vi "apply.vi"(8 "error in (no error)":errorcluster caption="entrée d'erreur (pas d'erreur)", 11 "Tree.lvclass 2":refnum<class "Tree.lvclass">) -> (0 "error out":errorcluster caption="sortie d'erreur", 2 "X_leaves":dbl[][](array[numeric]), 3 "Tree.lvclass":refnum<class "Tree.lvclass">)   [LabVIEW 2020, in "Tree.lvclass"]
doc: "Return the index of the leaf that each sample is predicted as.\n\n .. versionadded:: 0.17\n\n Parameters\n ----------\n X : {array-like, sparse matrix} of shape (n_samples, n_features)\n The input samples. Internally, it will be converted to\n ``dtype=np.float32`` and if a sparse matrix is provided\n to a sparse ``csr_matrix``.\n\n check_input : bool, default=True\n Allow to bypass several input checking.\n Don't use this parameter unless you know what you do.\n\n Returns\n -------\n X_leaves : array-like of shape (n_samples,)\n For each datapoint x in X, return the index of the leaf x\n ends up in. Leaves are numbered within\n ``[0; self.tree_.node_count)``, possibly with gaps in the\n numbering."
uses:
  Tree.lvclass
  C:/Users/cipop/TDF Dropbox/2_Technologies de France/1 - Services et Etudes/PLAIY/2 - DEV/PLAIYLAB/code/Python/Python.lvclass
  C:/Users/cipop/TDF Dropbox/2_Technologies de France/1 - Services et Etudes/PLAIY/2 - DEV/PLAIYLAB/code/Model/Model.lvclass
  Tree.lvclass/Tree.ctl
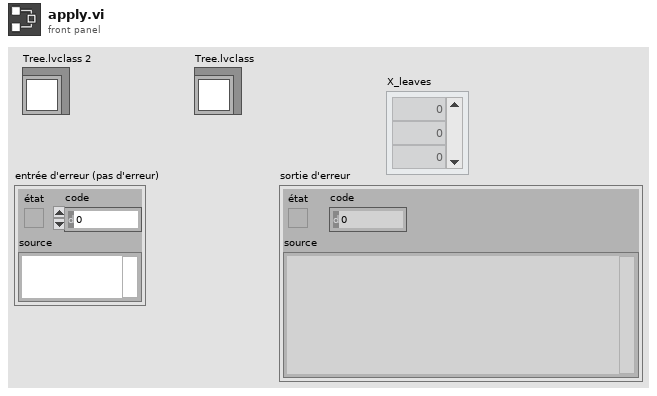
[diagram p1: front panel]
types:
  T1 = typedef "data.ctl" = cluster{"name":string, "X":dbl[][]}
  T2 = typedef "tree_data.ctl" = cluster{"y":dbl[][], "sample_weight":dbl[], "check_input":bool}
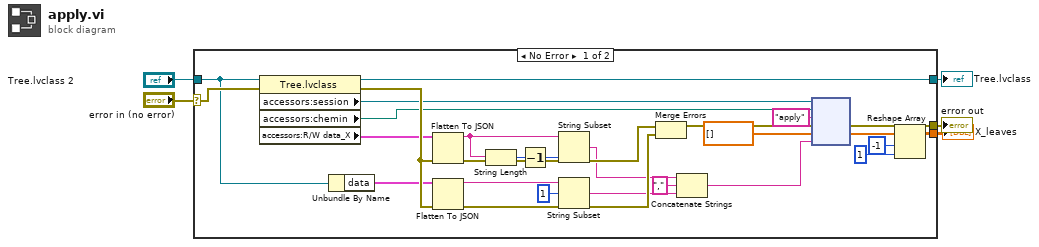
[diagram p0: block diagram]
diagram:
  n1 = case shown="No Error" "error in (no error)" {
    selector: "error in (no error)" -> [w30 w34]
    tunnel: [w31 w34] -> w4
    tunnel: [w13 w33] -> w2
    tunnel: "Tree.lvclass 2" -> [w12 w33]
    tunnel: [w8 _] -> w1
    frame No Error {
      n2 = property class="Tree.lvclass"(reference=w12, error in=w30) -> (reference out=w13:refnum<class "Tree.lvclass">, error out=w26:errorcluster, "accessors:session"=w16:refnum<k35>, "accessors:chemin"=w15:path, "accessors:R/W data_X"=w17:T1)
      n3 = Unbundle By Name(w12) -> ("data"=w11:T2)
      n4 = Flatten To JSON(anything=w17, error in (no error)=w26) -> (JSON string=w27:string, 11:w22:errorcluster)  [unwired: 1 in]
      n5 = Flatten To JSON(anything=w11, error in (no error)=w26) -> (JSON string=w24:string, 11:w23:errorcluster)  [unwired: 1 in]
      n6 = String Length(string=w27) -> (length=w29:i32)
      n7 = Decrement(x=w29) -> (x-1=w28:i32)
      n8 = String Subset(string=w27, length (rest)=w28) -> (substring=w20:string)  [unwired: 1 in]
      n9 = String Subset(string=w24, offset (0)=1) -> (substring=w19:string)  [unwired: 1 in]
      n10 = Merge Errors(w22, w23) -> (w14:errorcluster)
      n11 = Concatenate Strings(w20, "," ("string"), w19) -> (w18:string)
      n12 = node(w16, w15, "apply" ("nom de la fonction"), w14, dbl[] [], w18) -> (w31:errorcluster, w9:dbl[])  [unwired: 1 in, 3 out]
      n13 = Reshape Array(w9, -1 ("dimension size"), 1 ("dimension size")) -> (w8:dbl[][])
    }
    frame Error {
    }
  }
  "error out" <- w4
  "Tree.lvclass" <- w2
  "X_leaves" <- w1
